vi "Error Handler.vi"(8 "Error In":errorcluster) -> (0 "Error Out":errorcluster)   [LabVIEW 2019, in "Sequence Example.lvlib"]
uses:
  Sequence Example.lvlib
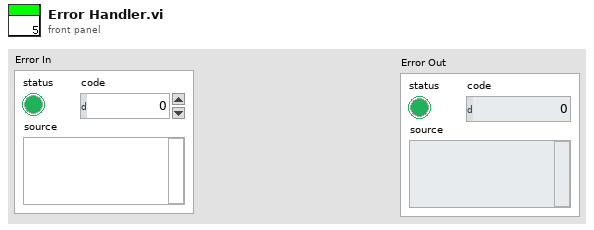
[diagram p1: front panel]
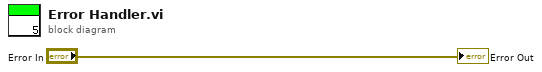
[diagram p0: block diagram]
diagram:
  "Error Out" <- "Error In"
